vi "Slop & Offset Data.vi"(10 "Input":T2(array[cluster])) -> (2 "Cluster":T1)   [LabVIEW 2015]
uses:
  <vilib>/Analysis/NI_AALPro.lvlib
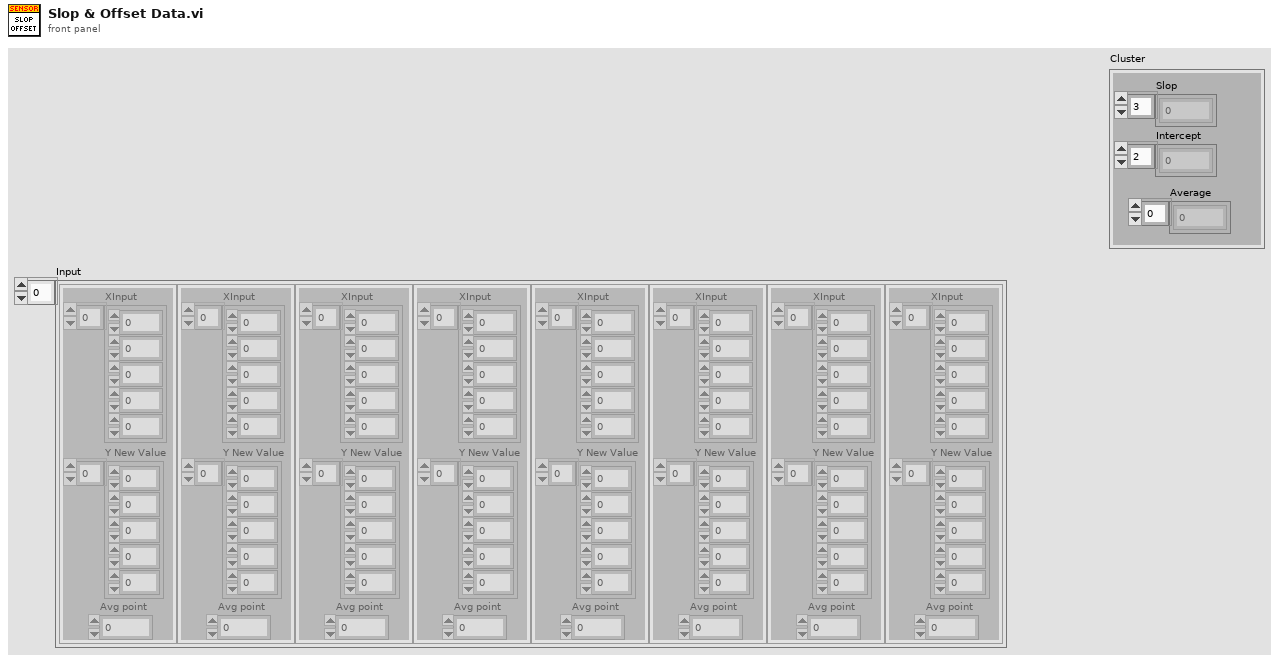
[diagram p1: front panel]
types:
  T1 = cluster{"Slop":dbl[], "Intercept":dbl[], "Average ":i16[]}
  T2 = cluster{"XInput":dbl[], "Y New Value":dbl[], "Avg point":i16}[]
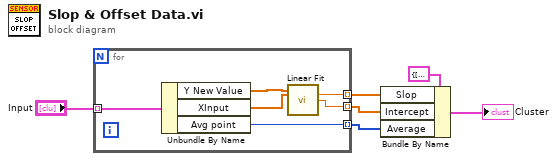
[diagram p0: block diagram]
diagram:
  n1 = for {
    tunnel: "Input" -> [w12] mode=indexing
    tunnel: [w9] -> w2 mode=indexing
    tunnel: [w8] -> w4 mode=indexing
    tunnel: [w7] -> w3 mode=indexing
    n2 = Unbundle By Name(w12) -> ("Y New Value"=w11:dbl[], "XInput"=w10:dbl[], "Avg point"=w9:i16)
    n3 = call <vilib>:"Linear Fit.vi"("Y"=w11, "X"=w10) -> ("slope"=w8:dbl, "intercept"=w7:dbl)  [unwired: 9 in, 3 out]
  }
  n4 = Bundle By Name(cluster=T1 {"Slop"=[], "Intercept"=[], "Average "=[]} ("Cluster 2"), "Slop"=w4, "Intercept"=w3, "Average"=w2) -> (→"Cluster":T1)
